vi "Read AE.vi"(8 "error in (no error)":errorcluster, 11 "CS++AEUpdate Msg in":refnum<class "CS++AEUpdate Msg.lvclass">) -> (0 "error out":errorcluster, 2 "AE":refnum<class "AE.lvclass">, 3 "CS++AEUpdate Msg out":refnum<class "CS++AEUpdate Msg.lvclass">)   [LabVIEW 2016, in "CS++PVMonitor.lvlib" / "CS++AEUpdate Msg.lvclass"]
doc: "Read attribute value."
uses:
  CS++AEUpdate Msg.lvclass
  Classes/CS++ProcessVariables/AlarmEvent/AE.lvclass
  CS++AEUpdate Msg.lvclass/CS++AEUpdate Msg.ctl
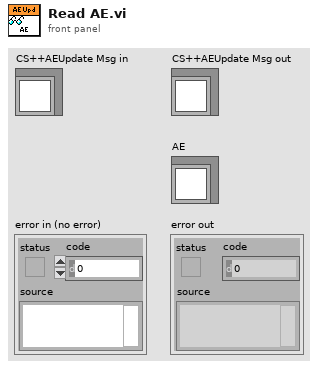
[diagram p1: front panel]
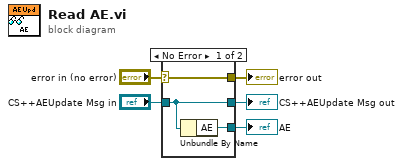
[diagram p0: block diagram]
diagram:
  n1 = case shown="No Error" "error in (no error)" {
    selector: "error in (no error)" -> [w8 w9]
    tunnel: [w8 w9] -> w4
    tunnel: [w7 w10] -> w1
    tunnel: "CS++AEUpdate Msg in" -> [w7 w10]
    tunnel: [w6 _] -> w2
    frame No Error {
      n2 = Unbundle By Name(w7) -> ("AE"=w6:refnum<class "AE.lvclass">)
    }
    frame Error {
    }
  }
  "error out" <- w4
  "CS++AEUpdate Msg out" <- w1
  "AE" <- w2
